vi "Disconnect.vi"(8 "error in (no error)":errorcluster, 11 "Oscilloscope in":refnum<class "Oscilloscope.lvclass">) -> (0 "error out":errorcluster, 3 "Oscilloscope out":refnum<class "Oscilloscope.lvclass">)   [LabVIEW 2018, in "Oscilloscope.lvlib" / "Oscilloscope.lvclass"]
doc: "This Override method is used finalize the communication session with the Oscope instrument."
uses:
  Oscilloscope.lvclass
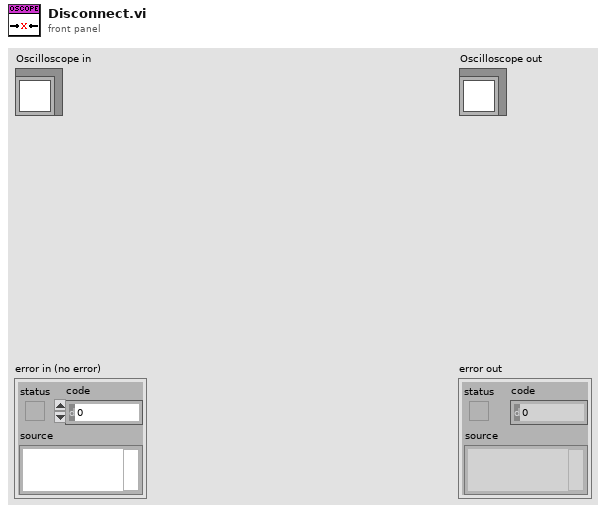
[diagram p1: front panel]
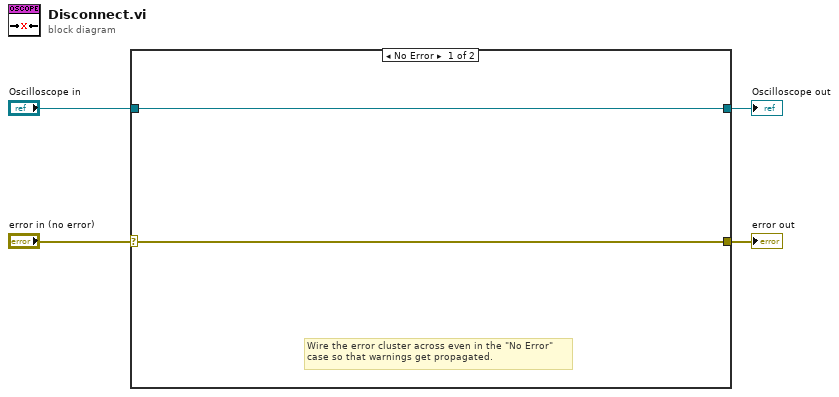
[diagram p0: block diagram]
diagram:
  n1 = case shown="No Error" "error in (no error)" {
    selector: "error in (no error)" -> [w5 w8]
    tunnel: [w5 w8] -> w3
    tunnel: [w6 w7] -> w1
    tunnel: "Oscilloscope in" -> [w6 w7]
    frame No Error {
      # "Wire the error cluster across even in the \"No Error\"\ncase so that warnings get propagated."
    }
    frame Error {
    }
  }
  "error out" <- w3
  "Oscilloscope out" <- w1
